vi "BMU诊断标定.vi"(8 "CAN端口":u16(ring), 9 "设备索引号":u16(ring), 10 "CAN卡类型":u32(ring)=21) -> ()   [LabVIEW 2013] (continued)
                                }
                                frame 4 {
                                }
                                }
                                n3193 = Reverse 1D Array(array=w4340) -> (reversed array=w4339:i32[])
                                n3194 = for {
                                N: w4335 -> [_]
                                tunnel: w4339 -> [w4357] mode=indexing
                                tunnel: [w4353] -> w4337 mode=indexing
                                n3195 = Equal To 0?(x=w4357) -> (x = 0?=w4356:bool)
                                n3196 = Select(t="无", s=w4356, f="故障") -> (s? t:f=w4353:string)
                                }
                                n3197 = Insert Into Array(array=w4338, new element=w4337) -> (w4336:string[])  [unwired: 1 in]
                              }
                              n3198 = call "详细故障分解.vi"("名称"=string[] ["自检异常(ee_cpu)", "存储空间满(ee_cpu)", "数据写入失败(ee_cpu)", "数据读取异常(ee_cpu)", "自检异常(ee_ext)", "存储空间满(ee_ext)", "数据写入失败(ee_ext)", "数据读取异常(ee_ext)", "自检异常(flash_ext)", "故障数据存储空间满(flash_ext)", "历史数据存储空间满(flash_ext)", "数据写入失败(flash_ext)", "数据读取失败(flash_ext)", "数据校验异常(flash_ext)", "自检异常(flash_cpu)", "存储空间满(flash_cpu)", "数据写入失败(flash_cpu)", "数据读取异常(flash_cpu)", "应用程序异常(cpu)", "应用程序下载异常(cpu)", "AD模块异常(cpu)", "RAM异常(cpu)", "CPU异常下电(cpu)"], "故障输入口"=w4330) -> ("输出数组"=w4328:string[][])  [unwired: 1 in, 2 out]
                              n3199 = local write "电池故障"(w4328) -> ()
                            }
                            frame 3 {
                              n3200 = for {
                                N: 5 -> [_]
                                tunnel: w4362 -> [w4379]
                                shift-right: [w4366] -> w4360
                                shift-left: string[] [] -> [w4368]
                                i -> [w4365]
                                w4373 = 8 ("索引")
                                w4377 = 2 ("y")
                                n3201 = Multiply(x=w4365, y=w4377) -> (x*y=w4378:i32)
                                n3202 = Array Subset(array=w4379, index=w4378, length=w4377) -> (w4376:u8[])
                                n3203 = Index Array(array=w4376) -> (element #1=w4375:u8, element #2=w4374:u8)  [unwired: 2 in]
                                n3204 = call "二进制解析-8.6.vi"("索引"=w4373, "数值"=w4375) -> ("低位子数组"=w4372:i32[])  [unwired: 1 in, 2 out]
                                n3205 = call "二进制解析-8.6.vi"("索引"=w4373, "数值"=w4374) -> ("低位子数组"=w4371:i32[])  [unwired: 1 in, 2 out]
                                n3206 = Insert Into Array(array=w4372, new element=w4371) -> (w4370:i32[])  [unwired: 1 in]
                                n3207 = Reverse 1D Array(array=w4370) -> (reversed array=w4369:i32[])
                                n3208 = for {
                                N: 6 -> [_]
                                tunnel: w4369 -> [w4384] mode=indexing
                                tunnel: [w4380] -> w4367 mode=indexing
                                n3209 = Equal To 0?(x=w4384) -> (x = 0?=w4383:bool)
                                n3210 = Select(t="无", s=w4383, f="故障") -> (s? t:f=w4380:string)
                                }
                                n3211 = Insert Into Array(array=w4368, new element=w4367) -> (w4366:string[])  [unwired: 1 in]
                              }
                              n3212 = call "详细故障分解.vi"("名称"=string[] ["初始化失败(CAN4)", "发送异常(CAN4)", "接收异常(CAN4)", "总线超时(CAN4)", "BUSOFF(CAN4)", "帧格式(CAN4)", "初始化异常(CAN0)", "发送异常(CAN0)", "接收异常(CAN0)", "总线超时(CAN0)", "BUSOFF(CAN0)", "帧格式(CAN0)", "初始化异常(CAN1)", "发送异常(CAN1)", "接收异常(CAN1)", "总线超时(CAN1)", "BUSOFF(CAN1)", "帧格式(CAN1)", "初始化失败(CAN2)", "发送异常(CAN2)", "接收异常(CAN2)", "总线超时(CAN2)", "BUSOFF(CAN2)", "帧格式(CAN2)", "初始化失败(CAN3)", "发送异常(CAN3)", "接收异常(CAN3)", "总线超时(CAN3)", "BUSOFF(CAN3)", "帧格式(CAN3)"], "故障输入口"=w4360) -> ("输出数组"=w4358:string[][])  [unwired: 1 in, 2 out]
                              n3213 = local write "电池故障"(w4358) -> ()
                            }
                            frame 4 {
                              n3214 = for {
                                N: 1 -> [_]
                                tunnel: w4389 -> [w4406]
                                shift-right: [w4393] -> w4387
                                shift-left: string[] [] -> [w4395]
                                i -> [w4392]
                                w4400 = 8 ("索引")
                                w4404 = 2 ("y")
                                n3215 = Multiply(x=w4392, y=w4404) -> (x*y=w4405:i32)
                                n3216 = Array Subset(array=w4406, index=w4405, length=w4404) -> (w4403:u8[])
                                n3217 = Index Array(array=w4403) -> (element #1=w4402:u8, element #2=w4401:u8)  [unwired: 2 in]
                                n3218 = call "二进制解析-8.6.vi"("索引"=w4400, "数值"=w4402) -> ("低位子数组"=w4399:i32[])  [unwired: 1 in, 2 out]
                                n3219 = call "二进制解析-8.6.vi"("索引"=w4400, "数值"=w4401) -> ("低位子数组"=w4398:i32[])  [unwired: 1 in, 2 out]
                                n3220 = Insert Into Array(array=w4399, new element=w4398) -> (w4397:i32[])  [unwired: 1 in]
                                n3221 = Reverse 1D Array(array=w4397) -> (reversed array=w4396:i32[])
                                n3222 = for {
                                N: 4 -> [_]
                                tunnel: w4396 -> [w4411] mode=indexing
                                tunnel: [w4407] -> w4394 mode=indexing
                                n3223 = Equal To 0?(x=w4411) -> (x = 0?=w4410:bool)
                                n3224 = Select(t="无", s=w4410, f="故障") -> (s? t:f=w4407:string)
                                }
                                n3225 = Insert Into Array(array=w4395, new element=w4394) -> (w4393:string[])  [unwired: 1 in]
                              }
                              n3226 = call "详细故障分解.vi"("名称"=string[] ["通讯协议版本不一致(soft)", "系统不同步(soft)", "软件版本不一致(soft)", "同硬件平台不兼容(soft)"], "故障输入口"=w4387) -> ("输出数组"=w4385:string[][])  [unwired: 1 in, 2 out]
                              n3227 = local write "电池故障"(w4385) -> ()
                            }
                            frame 5 {
                              n3228 = for {
                                N: 2 -> [_]
                                tunnel: w4416 -> [w4433]
                                shift-right: [w4420] -> w4414
                                shift-left: string[] [] -> [w4422]
                                i -> [w4419]
                                w4427 = 8 ("索引")
                                w4431 = 2 ("y")
                                n3229 = Multiply(x=w4419, y=w4431) -> (x*y=w4432:i32)
                                n3230 = Array Subset(array=w4433, index=w4432, length=w4431) -> (w4430:u8[])
                                n3231 = Index Array(array=w4430) -> (element #1=w4429:u8, element #2=w4428:u8)  [unwired: 2 in]
                                n3232 = call "二进制解析-8.6.vi"("索引"=w4427, "数值"=w4429) -> ("低位子数组"=w4426:i32[])  [unwired: 1 in, 2 out]
                                n3233 = call "二进制解析-8.6.vi"("索引"=w4427, "数值"=w4428) -> ("低位子数组"=w4425:i32[])  [unwired: 1 in, 2 out]
                                n3234 = Insert Into Array(array=w4426, new element=w4425) -> (w4424:i32[])  [unwired: 1 in]
                                n3235 = Reverse 1D Array(array=w4424) -> (reversed array=w4423:i32[])
                                n3236 = for {
                                N: 4 -> [_]
                                tunnel: w4423 -> [w4438] mode=indexing
                                tunnel: [w4434] -> w4421 mode=indexing
                                n3237 = Equal To 0?(x=w4438) -> (x = 0?=w4437:bool)
                                n3238 = Select(t="无", s=w4437, f="故障") -> (s? t:f=w4434:string)
                                }
                                n3239 = Insert Into Array(array=w4422, new element=w4421) -> (w4420:string[])  [unwired: 1 in]
                              }
                              n3240 = call "详细故障分解.vi"("名称"=string[] ["初始化失败(RS232)", "发送异常(RS232)", "接收异常(RS232)", "总线超时(RS232)", "初始化失败(RS485)", "发送异常(RS485)", "接收异常(RS485)", "总线超时(RS485)"], "故障输入口"=w4414) -> ("输出数组"=w4412:string[][])  [unwired: 1 in, 2 out]
                              n3241 = local write "电池故障"(w4412) -> ()
                            }
                            frame 6 {
                              n3242 = for {
                                N: 2 -> [_]
                                tunnel: w4443 -> [w4460]
                                shift-right: [w4447] -> w4441
                                shift-left: string[] [] -> [w4449]
                                i -> [w4446]
                                w4454 = 8 ("索引")
                                w4458 = 2 ("y")
                                n3243 = Multiply(x=w4446, y=w4458) -> (x*y=w4459:i32)
                                n3244 = Array Subset(array=w4460, index=w4459, length=w4458) -> (w4457:u8[])
                                n3245 = Index Array(array=w4457) -> (element #1=w4456:u8, element #2=w4455:u8)  [unwired: 2 in]
                                n3246 = call "二进制解析-8.6.vi"("索引"=w4454, "数值"=w4456) -> ("低位子数组"=w4453:i32[])  [unwired: 1 in, 2 out]
                                n3247 = call "二进制解析-8.6.vi"("索引"=w4454, "数值"=w4455) -> ("低位子数组"=w4452:i32[])  [unwired: 1 in, 2 out]
                                n3248 = Insert Into Array(array=w4453, new element=w4452) -> (w4451:i32[])  [unwired: 1 in]
                                n3249 = Reverse 1D Array(array=w4451) -> (reversed array=w4450:i32[])
                                n3250 = for {
                                N: 16 -> [_]
                                tunnel: w4450 -> [w4465] mode=indexing
                                tunnel: [w4461] -> w4448 mode=indexing
                                n3251 = Equal To 0?(x=w4465) -> (x = 0?=w4464:bool)
                                n3252 = Select(t="无", s=w4464, f="故障") -> (s? t:f=w4461:string)
                                }
                                n3253 = Insert Into Array(array=w4449, new element=w4448) -> (w4447:string[])  [unwired: 1 in]
                              }
                              n3254 = call "详细故障分解.vi"("名称"=string[] ["DI1对地短", "DI1对电源短", "DI2对地短", "DI2对电源短", "DI3对地短", "DI3对电源短", "DI4对地短", "DI4对电源短", "DI5对地短", "DI5对电源短", "DI6对地短", "DI6对电源短", "DI7对地短", "DI7对电源短", "DI8对地短", "DI8对电源短", "DO1对地短", "DO1对电源短", "DO2对地短", "DO2对电源短", "DO3对地短", "DO3对电源短", "DO4对地短", "DO4对电源短", "DO5对地短", "DO5对电源短", "DO6对地短", "DO6对电源短", "DO7对地短", "DO7对电源短", "DO8对地短", "DO8对电源短"], "故障输入口"=w4441) -> ("输出数组"=w4439:string[][])  [unwired: 1 in, 2 out]
                              n3255 = local write "电池故障"(w4439) -> ()
                            }
                            frame 7 {
                              n3256 = for {
                                N: 2 -> [_]
                                tunnel: w4470 -> [w4487]
                                shift-right: [w4474] -> w4468
                                shift-left: string[] [] -> [w4476]
                                i -> [w4472]
                                w4481 = 8 ("索引")
                                w4485 = 2 ("y")
                                n3257 = Multiply(x=w4472, y=w4485) -> (x*y=w4486:i32)
                                n3258 = Array Subset(array=w4487, index=w4486, length=w4485) -> (w4484:u8[])
                                n3259 = Index Array(array=w4484) -> (element #1=w4483:u8, element #2=w4482:u8)  [unwired: 2 in]
                                n3260 = call "二进制解析-8.6.vi"("索引"=w4481, "数值"=w4483) -> ("低位子数组"=w4480:i32[])  [unwired: 1 in, 2 out]
                                n3261 = call "二进制解析-8.6.vi"("索引"=w4481, "数值"=w4482) -> ("低位子数组"=w4479:i32[])  [unwired: 1 in, 2 out]
                                n3262 = Insert Into Array(array=w4480, new element=w4479) -> (w4478:i32[])  [unwired: 1 in]
                                n3263 = case shown="1" w4472 {
                                tunnel: [4 6] -> w4473
                                frame 0, Default {
                                }
                                frame 1 {
                                }
                                }
                                n3264 = Reverse 1D Array(array=w4478) -> (reversed array=w4477:i32[])
                                n3265 = for {
                                N: w4473 -> [_]
                                tunnel: w4477 -> [w4494] mode=indexing
                                tunnel: [w4490] -> w4475 mode=indexing
                                n3266 = Equal To 0?(x=w4494) -> (x = 0?=w4493:bool)
                                n3267 = Select(t="无", s=w4493, f="故障") -> (s? t:f=w4490:string)
                                }
                                n3268 = Insert Into Array(array=w4476, new element=w4475) -> (w4474:string[])  [unwired: 1 in]
                              }
                              n3269 = call "详细故障分解.vi"("名称"=string[] ["超时(pre-chg)", "后端开路(pre-chg)", "后端短路(pre-chg)", "预充电回路断开(pre-chg)", "正级继电器驱动故障(relay_driver)", "负级继电器驱动故障(relay_driver)", "预充电继电器驱动故障(relay_driver)", "充电继电器驱动故障(relay_driver)", "风机继电器驱动故障(relay_driver)", "加热继电器驱动故障(relay_driver)"], "故障输入口"=w4468) -> ("输出数组"=w4466:string[][])  [unwired: 1 in, 2 out]
                              n3270 = local write "电池故障"(w4466) -> ()
                            }
                          }
                        }
                        frame True {
                          n3271 = Index Array(array=w4498, index #1=0 ("索引"), index #2=1 ("索引")) -> (element #1=w4501:u8, element #2=w4502:u8)
                          n3272 = Join Numbers(hi=w4501, lo=w4502) -> ((hi.lo)=w4500:u16)
                          n3273 = Number To Hexadecimal String(2:w4500) -> (0:w4499:string)  [unwired: 1 out]
                          n3274 = Concatenate Strings("读取错误，代码： " ("字符串"), "0x" ("字符串"), w4499) -> (w4497:string)
                          n3275 = One Button Dialog(message=w4497, button name ("OK")="是" ("按钮名称（“确定”）")) -> ()  [unwired: 1 out]
                        }
                      }
                      n3276 = local write "消除"(FALSE ("消除")) -> ()
                      n3277 = global write "EV05全局变量1.vi" "流控帧 2"(FALSE ("流控帧 2")) -> ()
                      n3278 = local write "控制1"(FALSE ("控制1")) -> ()
                      n3279 = global write "EV05全局变量1.vi" "写入超时"(TRUE ("写入超时")) -> ()
                    }
                  }
                }
              }
            }
          }
        }
      }
      frame Error {
      }
    }
  }
  n3280 = case shown="无错误" w36 {
    tunnel: w30 -> [w4507 _]
    tunnel: w8 -> [w4506 _]
    frame No Error {
      n3281 = case shown="\"全部写入\"" "全部写入" {
        tunnel: w4507 -> [_ _ w4639 _ _ _ _ _ _ _ _ _ _ _ _]
        tunnel: w4506 -> [_ _ w4638 _ _ _ _ _ _ _ _ _ _ _ _]
        frame "假", Default {
          n3282 = local write "强制终止读写标记"(FALSE ("强制终止读写标记")) -> ()
        }
        frame "单个写入" {
          n3283 = local read "主从选择"() -> (w4516:enum32{"主板", "从板"})
          n3284 = case shown="\"从板\"" w4516 {
            tunnel: [w4527 w4542] -> w4513
            tunnel: [0.0 w4540] -> w4517
            tunnel: [_ w4541] -> w4515
            tunnel: [w4525 _] -> w4514
            frame "主板", Default {
              n3285 = stacked-sequence {
                tunnel: [_ w4539] -> w4525
                frame #0 {
                  n3286 = control-ref of="高压参数"() -> (w4530:refnum<vi>)
                  n3287 = control-ref of="电池信息"() -> (w4531:refnum<vi>)
                  n3288 = control-ref of="一级故障"() -> (w4537:refnum<vi>)
                  n3289 = control-ref of="一级故障 2"() -> (w4535:refnum<vi>)
                  n3290 = control-ref of="一级故障 3"() -> (w4534:refnum<vi>)
                  n3291 = control-ref of="加热控制参数"() -> (w4533:refnum<vi>)
                  n3292 = control-ref of="充电控制参数"() -> (w4532:refnum<vi>)
                  n3293 = control-ref of="项目信息"() -> (w4536:refnum<vi>)
                  n3294 = control-ref of="项目信息2"() -> (w4538:refnum<vi>)
                  n3295 = local read "主板数据"() -> (w4528:T4)
                  n3296 = Bundle(cluster=w4528, "项目信息"=w4536, "一级故障 4"=w4538, "一级故障"=w4537, "一级故障 2"=w4535, "一级故障 3"=w4534, "加热控制参数"=w4533, "充电控制参数"=w4532, "高压参数"=w4530, "电池信息"=w4531) -> (w4529:T4)
                  n3297 = local write "主板数据"(w4529) -> ()
                }
                frame #1 {
                  n3298 = control-ref of="主板数据"() -> (w4539:refnum<vi>)
                }
              }
              n3299 = local read "主板选项"() -> (w4527:string)
            }
            frame "从板" {
              n3300 = stacked-sequence {
                tunnel: [_ w4553] -> w4541
                frame #0 {
                  n3301 = control-ref of="从板号"() -> (w4552:refnum<vi>)
                  n3302 = control-ref of="项目信息 2"() -> (w4551:refnum<vi>)
                  n3303 = control-ref of="均衡参数"() -> (w4546:refnum<vi>)
                  n3304 = control-ref of="加热控制参数"() -> (w4550:refnum<vi>)
                  n3305 = control-ref of="一级故障(从板)"() -> (w4549:refnum<vi>)
                  n3306 = control-ref of="二级故障(从板)"() -> (w4548:refnum<vi>)
                  n3307 = control-ref of="三级故障(从板)"() -> (w4547:refnum<vi>)
                  n3308 = control-ref of="电池组信息"() -> (w4543:refnum<vi>)
                  n3309 = local read "从板信息"() -> (w4544:T2)
                  n3310 = Bundle(cluster=w4544, "从板号"=w4552, "项目信息 2"=w4551, "加热控制参数"=w4550, "一级故障(从板)"=w4549, "二级故障(从板)"=w4548, "三级故障(从板)"=w4547, "电池组信息(从板)"=w4543, "均衡参数"=w4546) -> (w4545:T2)
                  n3311 = local write "从板信息"(w4545) -> ()
                }
                frame #1 {
                  n3312 = control-ref of="从板信息"() -> (w4553:refnum<vi>)
                }
              }
              n3313 = local read "从板选项"() -> (w4542:string)
              n3314 = local read "从板号"() -> (w4540:u8)
            }
          }
          n3315 = local read "从板个数"() -> (w4518:dbl)
          n3316 = local read "快换"() -> (w4519:bool)
          n3317 = call "输入数据解析.vi"("单个参数补充"=w4518, "从板号"=w4517, "主板引用"=w4514, "从板引用"=w4515, "主板选项"=w4513, "枚举"=w4516, "快换"=w4519) -> ("输出数组"=w4523:dbl[][], "数组长度"=w4522:dbl[], "循环次数"=w4512:i32, "命令"=w4521:u32, "名称"=w4511:string[], "命令序号"=w4520:u32[])  [unwired: 2 in, 1 out]
          n3318 = for {
            N: w4512 -> [w4559]
            tunnel: w4523 -> [w4569]
            tunnel: w4522 -> [w4568]
            tunnel: w4521 -> [w4567]
            tunnel: w4520 -> [w4566]
            tunnel: w4517 -> [w4557]
            tunnel: w4513 -> [w4565]
            tunnel: w4511 -> [w4561]
            tunnel: [w4554] -> w4510
            i -> [w4560]
            n3319 = Index Array(array=w4569, index (row)=w4560) -> (element=w4564:dbl[])  [unwired: 1 in]
            n3320 = Index Array(array=w4568, index=w4560) -> (element=w4563:dbl)
            n3321 = Index Array(array=w4561, index=w4560) -> (element=w4558:string)
            n3322 = case shown="\"从板号\"" w4558 {
              tunnel: [w4571 w4572] -> w4556
              tunnel: w4557 -> [w4571 _]
              tunnel: [TRUE ("确定") w4573] -> w4555
              frame "假", Default {
              }
              frame "从板号" {
                n3323 = call "请输入当前从板板号"() -> ("当前从板板号"=w4572:dbl, "确定"=w4573:bool)  [unwired: 17 in, 1 out]
                n3324 = local write "当前从板板号"(w4572) -> ()
              }
            }
            n3325 = Index Array(array=w4566, index=w4560) -> (element=w4562:u32)
            n3326 = global write "全局 1.vi" "名称"(w4558) -> ()
            n3327 = case shown="真" w4555 {
              tunnel: w4567 -> [_ w4583]
              tunnel: w4565 -> [_ w4582]
              tunnel: w4564 -> [_ w4581]
              tunnel: w4563 -> [_ w4580]
              tunnel: w4562 -> [_ w4579]
              tunnel: w4560 -> [_ w4578]
              tunnel: w4558 -> [_ w4577]
              tunnel: w4559 -> [_ w4576]
              tunnel: w4556 -> [_ w4575]
              tunnel: [_ w4574] -> w4554
              frame False {
                n3328 = call <vilib>:"Unset Busy.vi"() -> ()  [unwired: 11 in, 1 out]
              }
              frame True {
                n3329 = stacked-sequence {
                  seq-local: [_ _ _ w4611 _ _] -> [_ _ _ _ w4620 _]
                  tunnel: w4581 -> [_ _ w4596 _ _ _]
                  tunnel: w4580 -> [_ _ w4595 _ _ _]
                  tunnel: w4583 -> [_ _ w4589 _ _ _]
                  tunnel: w4579 -> [_ _ w4587 _ _ _]
                  tunnel: w4582 -> [_ _ _ _ _ _]
                  tunnel: w4578 -> [_ _ _ _ _ w4631]
                  tunnel: w4577 -> [_ _ _ _ w4619 _]
                  tunnel: w4576 -> [_ _ _ _ _ w4632]
                  tunnel: w4575 -> [_ _ w4588 _ _ _]
                  tunnel: [_ _ _ _ _ w4629] -> w4574
                  frame #0 {
                    w4585 = FALSE ("流控帧")
                    w4584 = TRUE ("流控帧 2")
                    n3330 = global write "EV05全局变量1.vi" "读取超时"(w4585) -> ()
                    n3331 = global write "EV05全局变量1.vi" "流控帧"(w4585) -> ()
                    n3332 = local write "消除"(w4584) -> ()
                    n3333 = local write "控制1"(w4584) -> ()
                    n3334 = global write "EV05全局变量1.vi" "流控帧 2"(w4584) -> ()
                    n3335 = local write "写?"(w4584) -> ()
                  }
                  frame #1 {
                    n3336 = Wait Until Next ms Multiple(millisecond multiple=u32 50 ("毫秒倍数")) -> ()  [unwired: 1 out]
                  }
                  frame #2 {
                    n3337 = local read "设备索引号"() -> (w4591:u16)
                    n3338 = local read "CAN卡类型"() -> (w4592:u32)
                    n3339 = Increment(x=w4595) -> (x+1=w4594:dbl)
                    n3340 = local read "CAN端口"() -> (w4590:u16)
                    n3341 = local write "命令"(w4589) -> ()
                    n3342 = local write "命令序号"(w4587) -> ()
                    n3343 = Reshape Array(w4596, w4594) -> (w4593:dbl[])
                    n3344 = stacked-sequence {
                      tunnel: w4593 -> [_ w4610]
                      tunnel: w4592 -> [w4599 w4609]
                      tunnel: w4591 -> [w4598 w4608]
                      tunnel: w4590 -> [w4597 w4607]
                      tunnel: w4589 -> [_ w4606]
                      tunnel: w4588 -> [_ w4605]
                      tunnel: w4587 -> [_ w4604]
                      frame #0 {
                        n3345 = disable-structure shown="禁用" {
                          disable-tunnel: w4599 -> [w4602 _]
                          disable-tunnel: w4598 -> [w4601 _]
                          disable-tunnel: w4597 -> [w4600 _]
                          frame Disabled {
                            n3346 = dll-call lib="PTH1mabs FBluewave New EnergySVN_WorkBMS_Monitor_Bnet01trunk参数设置data\nkerneldlls\nusbcan.dll" fn="VCI_ClearBuffer"("DeviceType"=w4602, "DeviceInd"=w4601, "CANInd"=w4600) -> (error out=w4603:errorcluster)  [unwired: 4 in, 4 out]
                            n3347 = call <vilib>:"Clear Errors.vi"("error in (no error)"=w4603) -> ()  [unwired: 6 in, 1 out]
                          }
                          frame Enabled {
                          }
                        }
                      }
                      frame #1 {
                        n3348 = call "多帧发送机制(EV05).vi"("can卡类型"=w4609, "设备索引号"=w4608, "CAN端口"=w4607, "命令"=w4606, "板号"=w4605, "命令序号"=w4604, "输入数据"=w4610) -> ()  [unwired: 1 in, 12 out]
                      }
                    }
                  }
                  frame #3 {
                    n3349 = while {
                      tunnel: [w4613] -> w4611
                      i -> [w4617]
                      stop <- w4614 stop-if-true
                      n3350 = local read "强制终止读写标记"() -> (w4612:bool)
                      n3351 = global read "EV05全局变量1.vi" "读取超时"() -> (w4613:bool)
                      n3352 = Greater Or Equal?(x=w4617, y=30) -> (x >= y?=w4615:bool)
                      n3353 = Wait Until Next ms Multiple(millisecond multiple=u32 100 ("毫秒倍数")) -> ()  [unwired: 1 out]
                      n3354 = Compound Arithmetic op=OR(w4612, w4613, w4615) -> (w4614:bool)
                    }
                  }
                  frame #4 {
                    n3355 = case shown="假" w4620 {
                      tunnel: w4619 -> [w4621 w4627]
                      frame False {
                        n3356 = control-ref of="结果"() -> (w4625:refnum<vi>)
                        n3357 = Concatenate Strings(w4621, "       写入失败" ("字符串")) -> (w4624:string)
                        n3358 = Build Array(w4624) -> (w4623:string[])
                        n3359 = call "表格编辑.vi"("新元素/子数组"=w4623, "活动单元格:单元格背景色"=u32 16740749, "MCListbox引用句柄"=w4625) -> ()  [unwired: 9 out]
                      }
                      frame True {
                        n3360 = case shown="\"从板号\"" w4627 {
                          frame "假", Default {
                          }
                          frame "从板号" {
                            n3361 = local read "从板号"() -> (w4628:u8)
                            n3362 = local write "当前从板板号"(w4628) -> ()
                          }
                        }
                      }
                    }
                  }
                  frame #5 {
                    n3363 = Increment(x=w4631) -> (x+1=w4630:i32)
                    n3364 = Equal?(x=w4632, y=w4630) -> (x = y?=w4629:bool)
                    n3365 = case shown="真" w4629 {
                      frame False {
                      }
                      frame True {
                        n3366 = control-ref of="结果"() -> (w4636:refnum<vi>)
                        n3367 = Concatenate Strings("写入完成" ("字符串")) -> (w4635:string)
                        n3368 = Build Array(w4635) -> (w4634:string[])
                        n3369 = call "表格编辑.vi"("新元素/子数组"=w4634, "活动单元格:单元格背景色"=u32 21937, "MCListbox引用句柄"=w4636) -> ()  [unwired: 9 out]
                      }
                    }
                  }
                }
              }
            }
          }
          n3370 = stacked-sequence {
            tunnel: w4510 -> [_]
            frame #0 {
              n3371 = call <vilib>:"Unset Busy.vi"() -> ()  [unwired: 2 in, 10 out]
              n3372 = local write "强制终止读写标记"(FALSE ("强制停止")) -> ()
            }
          }
        }
        frame "全部写入" {
          n3373 = local read "主从选择"() -> (w4645:enum32{"主板", "从板"})
          n3374 = case shown="\"从板\"" w4645 {
            tunnel: [string[] ["项目信息", "一级故障阀值", "二级故障阀值", "三级故障阀值", "加热控制参数", "充电控制参数", "电池信息", "二维码"] string[] ["从板信息", "一级故障阀值", "二级故障阀值", "三级故障阀值", "二维码"]] -> w4642
            tunnel: [0.0 ("从板号") w4843] -> w4646
            tunnel: [w4827 _] -> w4644
            tunnel: [_ w4844] -> w4643
            tunnel: w4639 -> [_ w4843]
            frame "主板", Default {
              n3375 = stacked-sequence {
                tunnel: [_ w4841] -> w4827
                frame #0 {
                  n3376 = control-ref of="电池信息"() -> (w4833:refnum<vi>)
                  n3377 = control-ref of="高压参数"() -> (w4832:refnum<vi>)
                  n3378 = control-ref of="一级故障"() -> (w4835:refnum<vi>)
                  n3379 = control-ref of="一级故障 2"() -> (w4837:refnum<vi>)
                  n3380 = control-ref of="一级故障 3"() -> (w4838:refnum<vi>)
                  n3381 = control-ref of="加热控制参数"() -> (w4839:refnum<vi>)
                  n3382 = control-ref of="充电控制参数"() -> (w4840:refnum<vi>)
                  n3383 = control-ref of="项目信息"() -> (w4836:refnum<vi>)
                  n3384 = control-ref of="项目信息2"() -> (w4834:refnum<vi>)
                  n3385 = local read "主板数据"() -> (w4831:T4)
                  n3386 = Bundle(cluster=w4831, "项目信息"=w4836, "一级故障 4"=w4834, "一级故障"=w4835, "一级故障 2"=w4837, "一级故障 3"=w4838, "加热控制参数"=w4839, "充电控制参数"=w4840, "高压参数"=w4832, "电池信息"=w4833) -> (w4830:T4)
                  n3387 = local write "主板数据"(w4830) -> ()
                }
                frame #1 {
                  n3388 = control-ref of="主板数据"() -> (w4841:refnum<vi>)
                }
              }
            }
            frame "从板" {
              (unwired) "均衡参数"
              n3389 = stacked-sequence {
                tunnel: [_ w4856] -> w4844
                frame #0 {
                  n3390 = control-ref of="从板号"() -> (w4850:refnum<vi>)
                  n3391 = control-ref of="项目信息 2"() -> (w4851:refnum<vi>)
                  n3392 = control-ref of="均衡参数"() -> (w4848:refnum<vi>)
                  n3393 = control-ref of="加热控制参数"() -> (w4852:refnum<vi>)
                  n3394 = control-ref of="一级故障(从板)"() -> (w4853:refnum<vi>)
                  n3395 = control-ref of="二级故障(从板)"() -> (w4854:refnum<vi>)
                  n3396 = control-ref of="三级故障(从板)"() -> (w4855:refnum<vi>)
                  n3397 = control-ref of="电池组信息"() -> (w4849:refnum<vi>)
                  n3398 = local read "从板信息"() -> (w4847:T2)
                  n3399 = Bundle(cluster=w4847, "从板号"=w4850, "项目信息 2"=w4851, "加热控制参数"=w4852, "一级故障(从板)"=w4853, "二级故障(从板)"=w4854, "三级故障(从板)"=w4855, "电池组信息(从板)"=w4849, "均衡参数"=w4848) -> (w4846:T2)
                  n3400 = local write "从板信息"(w4846) -> ()
                }
                frame #1 {
                  n3401 = control-ref of="从板信息"() -> (w4856:refnum<vi>)
                }
              }
              n3402 = local write "从板号"(w4843) -> ()
              n3403 = local write "失败"(FALSE ("失败")) -> ()
            }
          }
          n3404 = Array Size(array=w4642) -> (size(s)=w4641:i32)
          n3405 = for {
            tunnel: w4645 -> [w4657]
            tunnel: w4646 -> [w4660]
            tunnel: w4644 -> [w4659]
            tunnel: w4643 -> [w4658]
            tunnel: w4641 -> [w4652]
            tunnel: [w4651] -> w4640
            tunnel: w4638 -> [w4650]
            tunnel: w4642 -> [w4648] mode=indexing
            i -> [w4653]
            n3406 = local read "二维码"() -> (w4647:string)
            n3407 = disable-structure shown="禁用" {
              disable-tunnel: w4657 -> [w4670 _]
              disable-tunnel: w4653 -> [w4669 _]
              disable-tunnel: w4652 -> [w4668 _]
              disable-tunnel: [w4666 _] -> w4651
              frame Disabled {
                n3408 = Increment(x=w4669) -> (x+1=w4667:i32)
                n3409 = Less Or Equal?(x=w4668, y=w4667) -> (x <= y?=w4666:bool)
                n3410 = case shown="\"从板\"" w4670 {
                  tunnel: w4669 -> [w4672 w4686]
                  frame "主板", Default {
                    n3411 = case shown="6" w4672 {
                      tunnel: [T8."项目信息" ("主从板") T8."一级故障阀值" ("主从板") T8."二级故障阀值" ("主从板") T8."三级故障阀值" ("主从板") T8."控制参数" ("主从板") T8."电池信息" ("主从板")] -> w4671
                      frame 0, Default {
                        n3412 = local write "1"(TRUE ("1")) -> ()
                      }
                      frame 1 {
                        n3413 = local write "1 2"(TRUE ("1 2")) -> ()
                      }
                      frame 2 {
                        n3414 = local write "1 3"(TRUE ("1 3")) -> ()
                      }
                      frame 3 {
                        n3415 = local write "1 4"(TRUE ("1 4")) -> ()
                      }
                      frame 4, 5 {
                        n3416 = local write "1 5"(TRUE ("1 5")) -> ()
                      }
                      frame 6 {
                        n3417 = local write "1 11"(TRUE ("1 11")) -> ()
                      }
                    }
                    n3418 = local write "主板2"(w4671) -> ()
                  }
                  frame "从板" {
                    n3419 = case shown="1" w4686 {
                      tunnel: [T21."从板信息" ("等级 2") T21."从板信息" ("等级 2") T21."一级故障阀值" ("等级 2") T21."二级故障阀值" ("等级 2") T21."三级故障阀值" ("等级 2") T21."快换参数" ("等级 2") T14."均衡参数" ("等级 2")] -> w4685
                      frame 99, Default {
                        n3420 = local write "1 6"(TRUE ("1 6")) -> ()
                      }
                      frame 0 {
                        n3421 = local write "1 6"(TRUE ("1 6")) -> ()
                      }
                      frame 1 {
                        n3422 = local write "1 7"(TRUE ("1 7")) -> ()
                      }
                      frame 2 {
                        n3423 = local write "1 8"(TRUE ("1 8")) -> ()
                      }
                      frame 3 {
                        n3424 = local write "1 9"(TRUE ("1 9")) -> ()
                      }
                      frame 4 {
                        n3425 = local write "1 10"(TRUE ("1 10")) -> ()
                      }
                      frame 5 {
                        n3426 = local write "1 12"(TRUE ("1 10")) -> ()
                      }
                    }
                    n3427 = local write "等级 2"(w4685) -> ()
                  }
                }
              }
              frame Enabled {
              }
            }
            n3428 = local read "从板个数"() -> (w4665:dbl)
            n3429 = local read "快换"() -> (w4656:bool)
            n3430 = call "输入数据解析.vi"("单个参数补充"=w4665, "从板号"=w4660, "从板二维码"=w4647, "主板引用"=w4659, "从板引用"=w4658, "主板选项"=w4648, "枚举"=w4657, "快换"=w4656) -> ("输出数组"=w4664:dbl[][], "数组长度"=w4663:dbl[], "循环次数"=w4655:i32, "命令"=w4662:u32, "名称"=w4654:string[], "命令序号"=w4661:u32[])  [unwired: 1 in, 1 out]
            n3431 = for {
              N: w4655 -> [w4706]
              tunnel: w4664 -> [w4716]
              tunnel: w4663 -> [w4715]
              tunnel: w4662 -> [w4714]
              tunnel: w4661 -> [w4712]
              tunnel: w4660 -> [w4713]
              tunnel: w4654 -> [w4709]
              tunnel: w4651 -> [w4704]
              tunnel: w4648 -> [w4703]
              tunnel: w4650 -> [w4702]
              i -> [w4705]
              n3432 = Index Array(array=w4716, index (row)=w4705) -> (element=w4711:dbl[])  [unwired: 1 in]
              n3433 = Index Array(array=w4715, index=w4705) -> (element=w4710:dbl)
              n3434 = Index Array(array=w4709, index=w4705) -> (element=w4707:string)
              n3435 = Index Array(array=w4712, index=w4705) -> (element=w4708:u32)
              n3436 = local write "重试次数"(u8 0 ("重试次数")) -> ()
              n3437 = while {
                tunnel: w4714 -> [w4728]
                tunnel: w4713 -> [w4727]
                tunnel: w4711 -> [w4726]
                tunnel: w4710 -> [w4725]
                tunnel: w4708 -> [w4724]
                tunnel: w4707 -> [w4723]
                tunnel: w4706 -> [w4722]
                tunnel: w4705 -> [w4721]
                tunnel: w4704 -> [w4720]
                tunnel: w4703 -> [w4719]
                tunnel: w4702 -> [w4718]
                stop <- w4717 stop-if-true
                # "用于重测"
                n3438 = stacked-sequence {
                  seq-local: [_ _ _ w4756 _ _] -> [_ _ _ _ w4774 _]
                  tunnel: w4726 -> [_ _ w4743 _ _ _]
                  tunnel: w4725 -> [_ _ w4742 _ _ _]
                  tunnel: w4728 -> [_ _ w4738 _ _ _]
                  tunnel: w4727 -> [_ _ w4733 _ _ _]
                  tunnel: w4724 -> [_ _ w4739 _ _ _]
                  tunnel: w4723 -> [_ _ w4732 w4755 w4773 _]
                  tunnel: w4722 -> [_ _ _ _ _ w4796]
                  tunnel: w4721 -> [_ _ _ _ _ w4795]
                  tunnel: w4720 -> [_ _ _ _ _ w4793]
                  tunnel: w4719 -> [_ _ _ _ _ _]
                  tunnel: w4718 -> [_ _ w4734 _ _ _]
                  tunnel: [_ _ _ _ w4772 _] -> w4717
                  frame #0 {
                    w4730 = FALSE ("流控帧")
                    w4729 = TRUE ("流控帧 2")
                    n3439 = global write "EV05全局变量1.vi" "读取超时"(w4730) -> ()
                    n3440 = global write "EV05全局变量1.vi" "流控帧"(w4730) -> ()
                    n3441 = local write "消除"(w4729) -> ()
                    n3442 = local write "控制1"(w4729) -> ()
                    n3443 = global write "EV05全局变量1.vi" "流控帧 2"(w4729) -> ()
                    n3444 = local write "写?"(w4729) -> ()
                  }
                  frame #1 {
                    n3445 = Wait Until Next ms Multiple(millisecond multiple=u32 50 ("毫秒倍数")) -> ()  [unwired: 1 out]
                  }
                  frame #2 {
                    n3446 = global write "全局 1.vi" "名称"(w4732) -> ()
                    n3447 = local write "命令"(w4738) -> ()
                    n3448 = Equal?(x=w4732, y="从板号") -> (x = y?=w4735:bool)
                    n3449 = Select(t=w4734, s=w4735, f=w4733) -> (s? t:f=w4737:dbl)
                    n3450 = local write "命令序号"(w4739) -> ()
                    n3451 = local read "CAN卡类型"() -> (w4746:u32)
                    n3452 = local read "设备索引号"() -> (w4745:u16)
                    n3453 = local read "CAN端口"() -> (w4744:u16)
                    n3454 = Increment(x=w4742) -> (x+1=w4740:dbl)
                    n3455 = Reshape Array(w4743, w4740) -> (w4741:dbl[])
                    n3456 = stacked-sequence {
                      tunnel: w4746 -> [_ w4754]
                      tunnel: w4745 -> [_ w4753]
                      tunnel: w4744 -> [_ w4752]
                      tunnel: w4741 -> [_ w4751]
                      tunnel: w4737 -> [_ w4750]
                      tunnel: w4739 -> [_ w4749]
                      tunnel: w4738 -> [_ w4748]
                      frame #0 {
                      }
                      frame #1 {
                        n3457 = call "多帧发送机制(EV05).vi"("can卡类型"=w4754, "设备索引号"=w4753, "CAN端口"=w4752, "命令"=w4748, "板号"=w4750, "命令序号"=w4749, "输入数据"=w4751) -> ("错误输出"=w4747:errorcluster)  [unwired: 1 in, 11 out]
                        n3458 = call <vilib>:"Clear Errors.vi"("error in (no error)"=w4747) -> ()  [unwired: 6 in, 1 out]
                      }
                    }
                    "Step" <- w4732
                  }
                  frame #3 {
                    n3459 = case shown="\"从板号\"" w4755 {
                      tunnel: [w4757 TRUE ("读取超时")] -> w4756
                      frame "假", Default {
                        n3460 = while {
                          tunnel: [w4759] -> w4757
                          i -> [w4764]
                          stop <- w4761 stop-if-true
                          n3461 = local read "强制终止读写标记"() -> (w4758:bool)
                          n3462 = global read "EV05全局变量1.vi" "读取超时"() -> (w4759:bool)
                          n3463 = Greater Or Equal?(x=w4764, y=30) -> (x >= y?=w4762:bool)
                          n3464 = Wait Until Next ms Multiple(millisecond multiple=u32 100 ("毫秒倍数")) -> ()  [unwired: 1 out]
                          n3465 = Compound Arithmetic op=OR(w4758, w4759, w4762) -> (w4761:bool)
                        }
                      }
                      frame "从板号" {
                        (unwired) u32 9 ("表格总行数")
                        (unwired) 5 ("保留行数")
                        n3466 = global read "全局 1.vi" "名称"() -> (w4770:string)
                        n3467 = control-ref of="结果"() -> (w4765:refnum<vi>)
                        n3468 = Concatenate Strings(w4770, "       写入成功" ("字符串")) -> (w4767:string)
                        n3469 = Build Array(w4767) -> (w4768:string[])
                        n3470 = call "表格编辑.vi"("新元素/子数组"=w4768, "活动单元格:单元格背景色"=u32 6618880, "MCListbox引用句柄"=w4765) -> ()  [unwired: 9 out]
                      }
                    }
                  }
                  frame #4 {
                    n3471 = case shown="假" w4774 {
                      tunnel: w4773 -> [w4776 _]
                      tunnel: [w4775 TRUE] -> w4772
                      frame False {
                        n3472 = local read "重试次数"() -> (w4780:u8)
                        n3473 = Increment(x=w4780) -> (x+1=w4779:u8)
                        n3474 = Greater Or Equal?(x=w4779, y=u8 4) -> (x >= y?=w4777:bool)
                        n3475 = local write "重试次数"(w4779) -> ()
                        n3476 = case shown="假" w4777 {
                          tunnel: w4776 -> [_ w4784]
                          tunnel: [FALSE TRUE] -> w4775
                          frame False {
                          }
                          frame True {
                            n3477 = control-ref of="结果"() -> (w4788:refnum<vi>)
                            n3478 = Concatenate Strings(w4784, "       写入失败" ("字符串")) -> (w4787:string)
                            n3479 = Build Array(w4787) -> (w4786:string[])
                            n3480 = call "表格编辑.vi"("新元素/子数组"=w4786, "活动单元格:单元格背景色"=u32 16740749, "MCListbox引用句柄"=w4788) -> ()  [unwired: 9 out]
                            "失败" <- TRUE
                          }
                        }
                      }
                      frame True {
                      }
                    }
                  }
                  frame #5 {
                    n3481 = Increment(x=w4795) -> (x+1=w4791:i32)
                    n3482 = Equal?(x=w4796, y=w4791) -> (x = y?=w4794:bool)
                    n3483 = And(x=w4793, y=w4794) -> (x .and. y?=w4792:bool)
                    n3484 = case shown="真" w4792 {
                      frame False {
                      }
                      frame True {
                        n3485 = Concatenate Strings("写入完成" ("字符串")) -> (w4799:string)
                        n3486 = control-ref of="结果"() -> (w4800:refnum<vi>)
                        n3487 = Build Array(w4799) -> (w4798:string[])
                        n3488 = call "表格编辑.vi"("新元素/子数组"=w4798, "活动单元格:单元格背景色"=u32 21937, "MCListbox引用句柄"=w4800) -> ()  [unwired: 9 out]
                      }
                    }
                  }
                }
              }
            }
            n3489 = local write "重试次数"(u8 0 ("重试次数")) -> ()
          }
          n3490 = stacked-sequence {
            tunnel: [_ w4813 _ _] -> _
            tunnel: w4640 -> [_ _ _ _]
            frame #0 {
              w4812 = "BMURESULT" ("section")
              n3491 = local read "失败"() -> (w4805:bool)
              n3492 = call <vilib>:"Open Config Data.vi"("error in (no error)"=errorcluster {"status"=FALSE, "code"=0, "source"=""}, "configuration file path"=path "D:/BlueWay/configresult.ini") -> ("error out"=w4810:errorcluster, "refnum"=w4807:T19)  [unwired: 7 in, 1 out]
              n3493 = Select(t="FAIL" ("key"), s=w4805, f="PASS" ("key")) -> (s? t:f=w4802:string)
              n3494 = call-poly <vilib>:"Write Key.vi"("section"=w4812, "error in (no error)"=w4810, "value"=w4802, "key"=w4812, "refnum"=w4807) -> ("error out"=w4811:errorcluster, "refnum out"=w4808:T19)  [unwired: 4 in, 1 out]
              n3495 = call <vilib>:"Close Config Data.vi"("error in (no error)"=w4811, "refnum"=w4808) -> ()  [unwired: 8 in, 2 out]
            }
            frame #1 {
              w4820 = u8 0 items=["Normal", "Listen Only"] ("工作方式")
              w4819 = u8 1 items=["Dual Filter", "Single Filter"] ("滤波方式")
              n3496 = local read "设备索引号"() -> (w4815:u16)
              n3497 = local read "CAN卡类型"() -> (w4814:u32)
              n3498 = local read "CAN端口"() -> (w4816:u16)
              n3499 = call "CAN_Init-8.6.vi"("CAN卡类型"=w4814, "设备索引号"=w4815, "CAN端口"=w4816, "操作类型"=enum16{"初始化CAN", "关闭CAN"}."关闭CAN", "滤波方式"=w4819, "Accept Code"=u32 3221225472, "簇"=T23 {"打开CAN"=FALSE, "初始化CAN"=FALSE, "开始CAN"=FALSE, "重启"=TRUE, "关闭CAN"=TRUE}, "Mask Code"=u32 1073741823 ("Accept Code"), "工作方式"=w4820, "是否滤波"=TRUE, "滤波选择"=T22 {"fiter_mode"=1, "fiter_endid"=402653184, "fiter_startid"=419430399}) -> ("error out"=w4813:errorcluster)  [unwired: 3 in, 5 out]
            }
            frame #2 {
              n3500 = Quit LabVIEW(quit? (T)=TRUE ("退出？(T)")) -> ()
            }
            frame #3 {
              n3501 = local write "停止"(TRUE ("停止")) -> ()
            }
          }
        }
        frame "单个读取" {
          n3502 = stacked-sequence {
            tunnel: [w4859] -> w4857
            frame #0 {
              n3503 = local read "主从选择"() -> (w4860:enum32{"主板", "从板"})
              n3504 = case shown="\"主板\", 默认" w4860 {
                tunnel: [w4873 w4953] -> w4862
                tunnel: [w4872 w4954] -> w4867
                tunnel: [0 ("从板号") w4950] -> w4866
                tunnel: [0 ("板号") u8 0 ("板号")] -> w4865
                tunnel: [w4868 w4949] -> w4863
                frame "主板", Default {
                  n3505 = local read "主板选项"() -> (w4869:string)
                  n3506 = case shown="\"SOC过低(3)\", \"SOC过高(3)\", \"SOH过低(3)\", \"充电电流过高(3)\", \"单体电压过低(3)\", \"单体电压过高(3)\", \"单组电压不均衡(3)\", \"单组温度不均衡(3)\", \"放电电流过高(3)\", \"极柱温度过高(3)\", \"内阻过大(3)\", \"三级故障阀值\", \"温度过低(3)\", \"温度过高(3)\", \"整组电压不均衡(3)\", \"整组温度不均衡(3)\", \"总电压过低(3)\", \"总电压过高(3)\"" w4869 {
                    tunnel: [_ u8[] [1, 2, 3, 4, 5, 6, 13, 8, 7, 9, 10, 11, 12] u8[] [1] u8[] [1] u8[] [2] u8[] [3] u8[] [4] u8[] [5] u8[] [6] u8[] [13] u8[] [7] u8[] [8] u8[] [9] u8[] [10] u8[] [14] u8[] [11] u8[] [12] u8[] [2] u8[] [3] u8[] [1] u8[] [2] u8[] [1] u8[] [2] u8[] [3] u8[] [4] u8[] [1, 2, 3, 4]] -> w4873
                    tunnel: [_ u8 128 ("命令") u8 129 ("命令") u8 128 ("命令") u8 128 ("命令") u8 128 ("命令") u8 128 ("命令") u8 128 ("命令") u8 128 ("命令") u8 128 ("命令") u8 128 ("命令") u8 128 ("命令") u8 128 ("命令") u8 128 ("命令") u8 128 ("命令") u8 128 ("命令") u8 128 ("命令") u8 129 ("命令") u8 129 ("命令") u8 130 ("命令") u8 130 ("命令") u8 132 ("命令") u8 132 ("命令") u8 132 ("命令") u8 132 ("命令") u8 132 ("命令")] -> w4872
                    tunnel: [_ string[] ["产品编号", "电压个数", "通道电压数", "电压起始值", "温度个数", "温度起始值", "保险位置", "电池额定实际容量", "SOC", "配置文件版本", "参数修改记录", "车牌号", "SOH"] string[] ["一级故障阀值"] string[] ["产品编号"] string[] ["电压个数"] string[] ["通道电压数"] string[] ["电压起始值"] string[] ["温度个数"] string[] ["温度起始值"] string[] ["保险位置"] string[] ["SOC"] string[] ["电池额定实际容量"] string[] ["配置文件版本"] string[] ["参数修改记录"] string[] ["校正时钟"] string[] ["车牌号"] string[] ["SOH"] string[] ["二级故障阀值"] string[] ["三级故障阀值"] string[] ["加热控制参数"] string[] ["充电控制参数"] string[] ["电池信息1"] string[] ["电池包组号"] string[] ["充放电安时"] string[] ["电池充放电次数"] string[] ["电池信息1", "电池包组号", "充放电安时", "电池充放电次数"]] -> w4868
                    frame "假", Default {
                    }
                    frame "项目信息" {
                    }
                    frame "SOC过低", "SOC过高", "SOH过低", "充电电流过高", "单体电压过低", "单体电压过高", "单组电压不均衡", "单组温度不均衡", "放电电流过高", "极柱温度过高", "内阻过大", "温度过低", "温度过高", "一级故障阀值", "整组电压不均衡", "整组温度不均衡", "总电压过低", "总电压过高" {
                    }
                    frame "产品编号" {
                    }
                    frame "电压个数" {
                    }
                    frame "通道电压数" {
                    }
                    frame "电压起始值" {
                    }
                    frame "温度个数" {
                    }
                    frame "温度起始值" {
                    }
                    frame "保险位置" {
                    }
                    frame "SOC" {
                    }
                    frame "电池额定实际容量" {
                    }
                    frame "配置文件版本" {
                    }
                    frame "参数修改记录" {
                    }
                    frame "校正时钟" {
                    }
                    frame "车牌号" {
                    }
                    frame "SOH" {
                    }
                    frame "SOC过低(2)", "SOC过高(2)", "SOH过低(2)", "充电电流过高(2)", "单体电压过低(2)", "单体电压过高(2)", "单组电压不均衡(2)", "单组温度不均衡(2)", "二级故障阀值", "放电电流过高(2)", "极柱温度过高(2)", "内阻过大(2)", "温度过低(2)", "温度过高(2)", "整组电压不均衡(2)", "整组温度不均衡(2)", "总电压过低(2)", "总电压过高(2)" {
                    }
                    frame "SOC过低(3)", "SOC过高(3)", "SOH过低(3)", "充电电流过高(3)", "单体电压过低(3)", "单体电压过高(3)", "单组电压不均衡(3)", "单组温度不均衡(3)", "放电电流过高(3)", "极柱温度过高(3)", "内阻过大(3)", "三级故障阀值", "温度过低(3)", "温度过高(3)", "整组电压不均衡(3)", "整组温度不均衡(3)", "总电压过低(3)", "总电压过高(3)" {
                    }
                    frame "风机关闭温差", "风机关闭温度", "风机开启温差", "风机开启温度", "加热关闭温差", "加热关闭温度", "加热开启温度", "加热控制参数" {
                    }
                    frame "充电控制参数", "电流步长", "最大允许充电电流", "最大允许充电温度", "最大允许单体电压", "最大允许总电压", "最小允许充电电流", "最小允许充电温度", "最小允许单体电压" {
                    }
                    frame "电池信息1" {
                    }
                    frame "电池包组号" {
                    }
                    frame "充放电安时" {
                    }
                    frame "电池充放电次数" {
                    }
                    frame "电池信息" {
                    }
                  }
                }
                frame "从板" {
                  n3507 = local read "从板选项"() -> (w4951:string)
                  n3508 = case shown="\"从板信息\"" w4951 {
                    tunnel: [_ u8 0 ("命令") u8 0 ("命令") u8 0 ("命令") u8 0 ("命令") u8 0 ("命令") u8 0 ("命令") u8 0 ("命令") u8 2 ("命令") u8 2 ("命令") u8 2 ("命令") u8 3 ("命令") u8 6 ("命令") u8 6 ("命令") u8 6 ("命令") u8 3 ("命令") u8 3 ("命令") u8 3 ("命令") u8 3 ("命令") u8 3 ("命令") u8 3 ("命令") u8 3 ("命令")] -> w4954
                    tunnel: [_ u8[] [6] u8[] [6, 1, 2, 3, 4, 5] u8[] [1] u8[] [2] u8[] [3] u8[] [4] u8[] [5] u8[] [1] u8[] [2] u8[] [3] u8[] [1, 2, 3, 4, 5, 6, 7] u8[] [1, 2] u8[] [2] u8[] [1] u8[] [1] u8[] [2] u8[] [3] u8[] [4] u8[] [5] u8[] [6] u8[] [7]] -> w4953
                    tunnel: [_ string[] ["从板号"] string[] ["从板号", "电压起始值", "通道电压个数", "保险位置", "温度起始值", "加热控制参数"] string[] ["电压起始值"] string[] ["通道电压节数"] string[] ["保险位置"] string[] ["温度起始值"] string[] ["加热控制参数"] string[] ["一级故障阀值"] string[] ["二级故障阀值"] string[] ["三级故障阀值"] string[] ["电池包信息1", "电池包序号", "充放电安时", "充电次数时间", "SOC", "车牌号", "充电参数"] string[] ["均衡阀值", "充电结束电压"] string[] ["充电结束电压"] string[] ["均衡阀值"] string[] ["电池包信息1"] string[] ["电池包序号"] string[] ["充放电安时"] string[] ["充电次数时间"] string[] ["SOC"] string[] ["车牌号"] string[] ["充电参数"]] -> w4949
                    frame "假", Default {
                    }
                    frame "从板号" {
                    }
                    frame "从板信息" {
                    }
                    frame "电压个数" {
                    }
                    frame "通道电压节数" {
                    }
                    frame "保险位置" {
                    }
                    frame "温度个数" {
                    }
                    frame "风机关闭温差", "风机关闭温度", "风机开启温差", "风机开启温度", "加热关闭温差", "加热关闭温度", "加热开启温度", "加热控制参数" {
                    }
                    frame "SOC过低", "电压不均衡", "电压过低", "电压过高", "温度不均衡", "温度过低", "温度过高", "一级故障阀值" {
                    }
                    frame "SOC过低(2)", "电压不均衡(2)", "电压过低(2)", "电压过高(2)", "二级故障阀值", "温度不均衡(2)", "温度过低(2)", "温度过高(2)" {
                    }
                    frame "SOC过低(3)", "电压不均衡(3)", "电压过低(3)", "电压过高(3)", "三级故障阀值", "温度不均衡(3)", "温度过低(3)", "温度过高(3)" {
                    }
                    frame "快换参数" {
                    }
                    frame "均衡参数" {
                    }
                    frame "充电结束电压" {
                    }
                    frame "均衡阀值" {
                    }
                    frame "电池包信息1" {
                    }
                    frame "电池包序号" {
                    }
                    frame "充放电安时" {
                    }
                    frame "充电次数时间" {
                    }
                    frame "SOC" {
                    }
                    frame "车牌号" {
                    }
                    frame "充电参数" {
                    }
                  }
                  n3509 = local read "从板号"() -> (w4950:u8)
                }
              }
              n3510 = Build Array(w4865) -> (w4864:i32[])
              n3511 = local write "命令"(w4867) -> ()
              n3512 = Array Size(array=w4862) -> (size(s)=w4861:i32)
              n3513 = for {
                tunnel: w4862 -> [w5026] mode=indexing
                tunnel: w4867 -> [w5025]
                tunnel: w4866 -> [w5024]
                tunnel: w4864 -> [w5023]
                tunnel: w4863 -> [w5022] mode=indexing
                tunnel: w4861 -> [w5021]
                tunnel: w4860 -> [w5019]
                tunnel: [w5018] -> w4859
                i -> [w5020]
                n3514 = while {
                  tunnel: w5026 -> [w5035]
                  tunnel: w5025 -> [w5034]
                  tunnel: w5024 -> [w5033]
                  tunnel: w5023 -> [w5032]
                  tunnel: w5022 -> [w5031]
                  tunnel: w5021 -> [w5030]
                  tunnel: w5020 -> [w5029]
                  tunnel: w5019 -> [w5028]
                  tunnel: [w5027] -> w5018
                  stop <- w5027 stop-if-true
                  n3515 = stacked-sequence {
                    seq-local: [_ _ _ _ w5183 _ _] -> [_ _ _ _ _ w5192 _]
                    tunnel: w5035 -> [_ _ _ w5171 _ _ _]
                    tunnel: w5034 -> [_ _ _ w5170 _ _ _]
                    tunnel: w5033 -> [_ _ _ w5169 _ _ _]
                    tunnel: w5032 -> [_ _ _ w5168 _ _ _]
                    tunnel: [_ _ _ _ w5184 _ _] -> w5027
                    tunnel: w5031 -> [w5037 _ _ _ _ w5193 _]
                    tunnel: w5030 -> [_ _ _ _ _ _ w5203]
                    tunnel: w5029 -> [_ _ _ _ _ _ w5202]
                    tunnel: w5028 -> [w5036 _ _ _ _ _ _]
                    frame #0 {
                      n3516 = case shown="\"主板\", 默认" w5036 {
                        tunnel: w5037 -> [w5038 w5129]
                        frame "主板", Default {
                          n3517 = case shown="\"电压个数\"" w5038 {
                            frame "假", Default {
                            }
                            frame "产品编号" {
                              n3518 = control-ref of="产品编号"() -> (w5040:refnum<vi>)
                              n3519 = property class="Str"(reference=w5040, "Value"="") -> ()  [unwired: 1 in, 2 out]
                            }
                            frame "电压个数" {
                              n3520 = local read "从板个数"() -> (w5041:dbl)
                              n3521 = control-ref of="项目信息"() -> (w5045:refnum<vi>)
                              n3522 = for {
                                N: w5041 -> [_]
                                tunnel: [""] -> w5044 mode=indexing
                              }
                              n3523 = call "表格数据输入-8.6.vi"("行数"=u32 0, "列数"=u32 1, "字符串数组"=w5044, "表格引用"=w5045) -> ()  [unwired: 8 in]
                            }
                            frame "通道电压数" {
                              n3524 = control-ref of="项目信息"() -> (w5051:refnum<vi>)
                              n3525 = for {
                                N: 20 -> [_]
                                tunnel: [""] -> w5050 mode=indexing
                              }
                              n3526 = local read "从板个数"() -> (w5052:dbl)
                              n3527 = Increment(x=w5052) -> (x+1=w5048:dbl)
                              n3528 = call "表格数据输入-8.6.vi"("行数"=w5048, "列数"=u32 1, "字符串数组"=w5050, "表格引用"=w5051) -> ()  [unwired: 8 in]
                            }
                            frame "电压起始值" {
                              n3529 = local read "从板个数"() -> (w5056:dbl)
                              n3530 = Increment(x=w5056) -> (x+1=w5055:dbl)
